vi "convertClusterToObject.vi"(0 "clusterData":variant, 1 "error in":errorcluster, 8 "objectType":refnum<class>) -> (14 "object out":refnum<class>, 15 "error out":errorcluster)   [LabVIEW 2020, in "JKI JSON Object Serialization.lvlib" / "OOP_Utility.lvlib"]
doc: "Transform a cluster to an object, applying cluster element values to class private data elements that have matching names.\n\nGCraftsman JSON Object Serialization Toolkit\nwww.GCraftsman.com\nCopyright (c) 2017, GCraftsman"
uses:
  OOP_Utility.lvlib
  Reflection/getClassHierarchyVersions.vi
  <vilib>/Utility/LVClass/Get LV Class Name.vi
  Reflection/reflectionPool.vi
  Reflection/Reflection.lvclass
  <vilib>/Utility/Data Type/NI_Data Type.lvlib
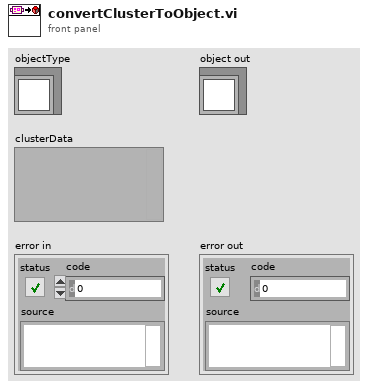
[diagram p1: front panel]
types:
  T1 = typedef "NI_Data Type.lvlib/Data Type.ctl" = enum8{"Invalid Type", "Void", "I8", "I16", "I32", "I64", "U8", "U16", "U32", "U64", "Single Float", "Double Float", "Extended Float", "Single Complex", "Double Complex", "Extended Complex", "Enum U8", "Enum U16", "Enum U32", "Enum U64", "Single Float With Unit", "Double Float With Unit", "Extended Float With Unit", "Single Complex with Unit", "Double Complex with Unit", "Extended Complex with Unit", "Boolean", "String", "Path", "Picture", "Tag", "Array", "Cluster", "Variant", "LV Variant", "Waveform", "Timestamp", "Digital Waveform", "Digital Data", "ExpressData", "Refnum", "External Data", "VI", "Poly VI", "LabVIEW Class Instance", "Fixed Point", "Set Collection", "Map Collection"}
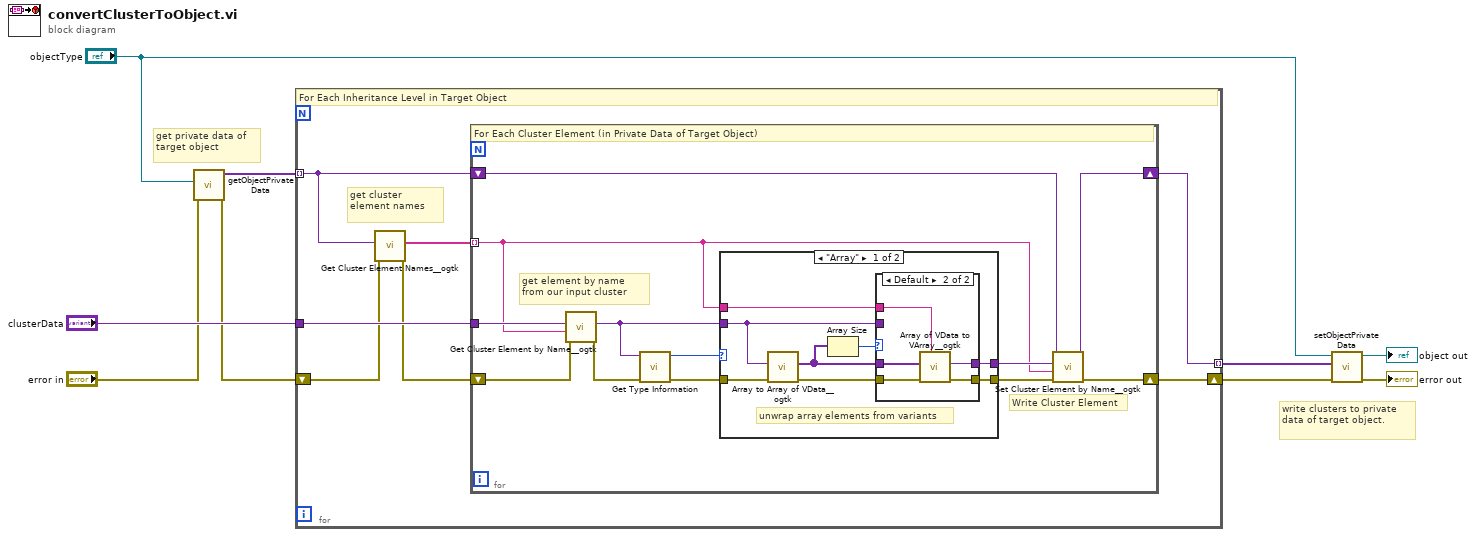
[diagram p0: block diagram]
diagram:
  # "write clusters to private data of target object."
  # "get private data of target object"
  n1 = call "getObjectPrivateData.vi"("error in (no error)"="error in", "object in"="objectType") -> ("error out"=w1:errorcluster, "private data"=w5:variant[])  [unwired: 6 in, 2 out]
  n2 = for {
    tunnel: w5 -> [w14] mode=indexing
    tunnel: "clusterData" -> [w16]
    tunnel: [w15] -> w7 mode=indexing
    shift-right: [w10] -> w8
    shift-left: w1 -> [w12]
    # "get cluster element names"
    # "For Each Inheritance Level in Target Object"
    n3 = call <userlib>:"Get Cluster Element Names__ogtk.vi"("error in (no error)"=w12, "Cluster"=w14) -> ("error out"=w11:errorcluster, "Element Names"=w13:string[])  [unwired: 8 in]
    n4 = for {
      tunnel: w16 -> [w28]
      shift-right: [w27] -> w15
      shift-left: w14 -> [w24]
      tunnel: w13 -> [w17] mode=indexing
      shift-right: [w25] -> w10
      shift-left: w11 -> [w26]
      # "Write Cluster Element"
      # "get element by name from our input cluster"
      # "For Each Cluster Element (in Private Data of Target Object)"
      n5 = call <userlib>:"Get Cluster Element by Name__ogtk.vi"("error in (no error)"=w26, "Element Name"=w17, "Cluster"=w28) -> ("error out"=w20:errorcluster, "VElement"=w21:variant)  [unwired: 6 in, 1 out]
      n6 = call <vilib>:"Get Type Information.vi"("error in (no error)"=w20, "variant"=w21) -> ("error out"=w19:errorcluster, "type"=w23:T1)  [unwired: 5 in, 3 out]
      n7 = case shown="\"Array\"" w23 {
        tunnel: [w35 w45] -> w22
        tunnel: w21 -> [w29 w45]
        tunnel: w19 -> [w36 w44]
        tunnel: [w33 w44] -> w18
        tunnel: w17 -> [w32 _]
        frame "Array" {
          # "unwrap array elements from variants"
          n8 = call <userlib>:"Array to Array of VData__ogtk.vi"("error in (no error)"=w36, "MultiD Array"=w29) -> ("error out"=w34:errorcluster, "1D Array of Variants"=w31:variant[])  [unwired: 8 in]
          n9 = Array Size(array=w31) -> (size(s)=w30:i32)
          n10 = case shown="Default" w30 {
            tunnel: [w37 w43] -> w35
            tunnel: w34 -> [w38 w42]
            tunnel: [w38 w41] -> w33
            tunnel: w32 -> [_ w40]
            tunnel: w31 -> [_ w39]
            tunnel: w29 -> [w37 _]
            frame 0 {
            }
            frame Default {
              n11 = call <userlib>:"Array of VData to VArray__ogtk.vi"("Array Name"=w40, "error in (no error)"=w42, "1D Array of VData"=w39) -> ("error out"=w41:errorcluster, "VArray"=w43:variant)  [unwired: 7 in]
            }
          }
        }
        frame Default {
        }
      }
      n12 = call <userlib>:"Set Cluster Element by Name__ogtk.vi"("error in (no error)"=w18, "Element Name (\"\": New Element Data Name)"=w17, "New Element Value"=w22, "Cluster"=w24) -> ("error out"=w25:errorcluster, "VCluster out"=w27:variant)  [unwired: 5 in, 1 out]
    }
  }
  n13 = call "setObjectPrivateData.vi"("error in (no error)"=w8, "privateData"=w7, "object in"="objectType") -> ("error out"=→"error out":errorcluster, "object out"=→"object out":refnum<class>)  [unwired: 6 in]
